vi "OFBS_saveResults.vi"(9 "Solution":i32[][][](array[numeric]), 10 "Accuracy Chart":cluster{i32[], dbl[]}[](graph), 11 "Optimization Algorithm":T1) -> (0 "error out":errorcluster, 3 "Results out":dbl[](array[numeric]))   [LabVIEW 2016, in "Optimal Frequency Bands Search.lvlib"]
doc: "Найти значения начальных границ и длин частотных диапазонов, для которых оценка точности классификации принимает максимальное значение. Сохранить полученное решение в текстовых файл. В названии файла указывается метод оптимизации и время создания."
uses:
  OFBS_AlgorithmTypes.ctl
  Optimal Frequency Bands Search.lvlib
panel:
  # "This VI is a part of BCI Design library, http://www.ru-bci.org \nCopyright © 2020, Sotnikov Peter, All rights reserved. License: GNU GPLv3"
  # "Sotnikov P (c), 2016"
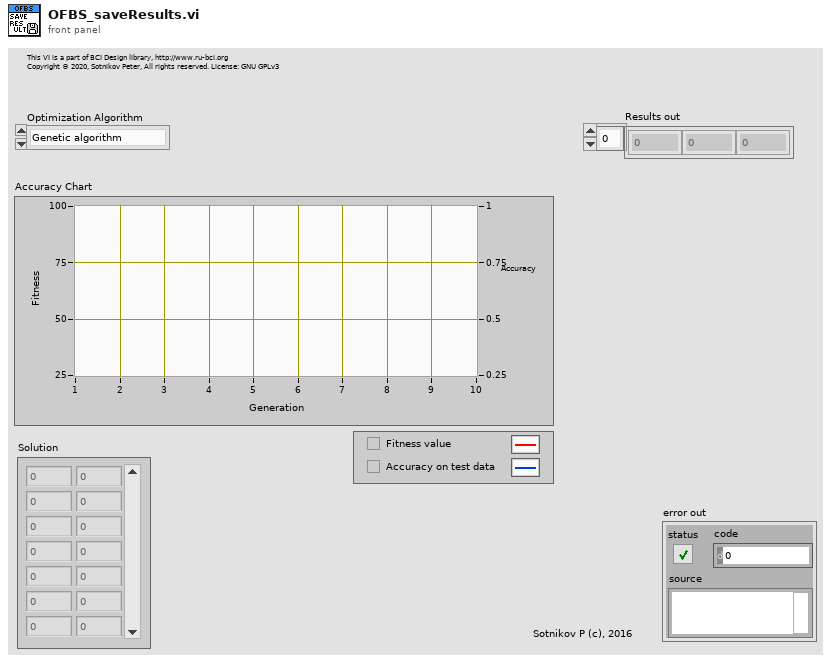
[diagram p1: front panel]
types:
  T1 = typedef "Optimal Frequency Bands Search.lvlib/OFBS_AlgorithmTypes.ctl" = enum16{"Genetic algorithm", "Particle swarm optimization"}
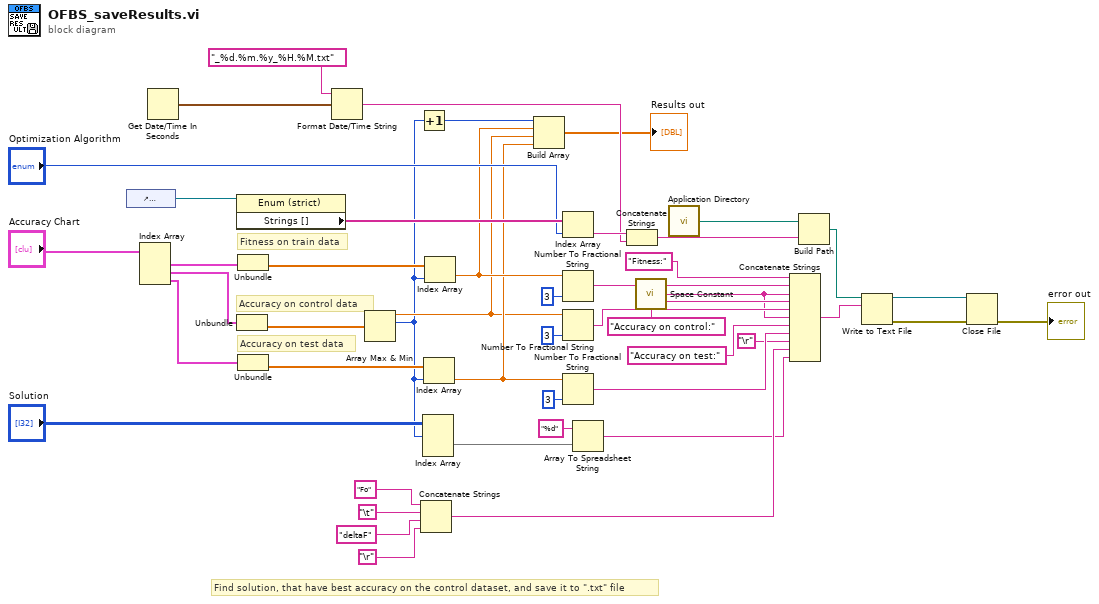
[diagram p0: block diagram]
diagram:
  # "Accuracy on test data"
  # "Find solution, that have best accuracy on the control dataset, and save it to \".txt\" file"
  # "Accuracy on control data"
  # "Fitness on train data"
  n1 = control-ref of="Optimization Algorithm"() -> (w18:refnum<vi>)
  n2 = Index Array "Index Array"(array="Accuracy Chart") -> (element #1=w46:cluster{i32[], dbl[]}, element #2=w47:cluster{i32[], dbl[]}, element #3=w16:cluster{i32[], dbl[]})  [unwired: 3 in]
  n3 = Get Date/Time In Seconds() -> (seconds since 1Jan1904=w37:timestamp)
  n4 = property on="Property Node" class="Enum (strict)"(reference=w18) -> ("Strings []"=w39:string[])  [unwired: 1 in, 2 out]
  n5 = Unbundle(w47) -> (w4:dbl[])  [unwired: 1 out]
  n6 = Unbundle(w46) -> (w45:dbl[])  [unwired: 1 out]
  n7 = Unbundle(w16) -> (w5:dbl[])  [unwired: 1 out]
  n8 = Format Date/Time String(time format string (%c)="_%d.%m.%y_%H.%M.txt", seconds (now)=w37) -> (date/time string=w35:string)  [unwired: 1 in]
  n9 = Array Max & Min(array=w4) -> (max value=w3:dbl, max index (indices)=w2:i32)  [unwired: 2 out]
  n10 = Increment(x=w2) -> (x+1=w1:i32)
  n11 = Concatenate Strings "Concatenate Strings"("Fo" ("string"), "\t", "deltaF" ("string"), "\r") -> (w10:string)
  n12 = Index Array(array="Solution", index (dim 0)=w2) -> (element=w44:i32[][])  [unwired: 2 in]
  n13 = Index Array(array=w5, index=w2) -> (element=w7:dbl)
  n14 = Index Array(array=w45, index=w2) -> (element=w8:dbl)
  n15 = Build Array(w1, w8, w3, w7) -> (→"Results out":dbl[])
  n16 = Index Array(array=w39, index="Optimization Algorithm") -> (element=w36:string)
  n17 = Number To Fractional String(number=w8, precision (6)=i16 3) -> (F-format string=w31:string)  [unwired: 2 in]
  n18 = Number To Fractional String(number=w3, precision (6)=i16 3) -> (F-format string=w29:string)  [unwired: 2 in]
  n19 = Number To Fractional String(number=w7, precision (6)=i16 3) -> (F-format string=w12:string)  [unwired: 2 in]
  n20 = Array To Spreadsheet String(array=w44, 3:"%d" ("format string")) -> (spreadsheet string=w9:string)  [unwired: 1 in]
  n21 = Concatenate Strings(w36, w35) -> (w34:string)
  n22 = call <vilib>:"Space Constant.vi"() -> ("String"=w14:string)
  n23 = call <vilib>:"Application Directory.vi"() -> ("Application Directory"=w38:path)
  n24 = Concatenate Strings("Fitness:" ("string"), w31, w14, "Accuracy on control:" ("string"), w29, w14, "Accuracy on test:" ("string"), w12, "\r", w10, w9) -> (w40:string)
  n25 = Build Path(base path=w38, name or relative path=w34) -> (appended path=w33:path)
  n26 = Write to Text File(file (use dialog)=w33, text=w40) -> (refnum out=w28:refnum<file>, error out=w27:errorcluster)  [unwired: 2 in, 1 out]
  n27 = Close File(refnum=w28, error in=w27) -> (error out=→"error out":errorcluster)  [unwired: 1 out]
